vi "End Map.vi"   [LabVIEW 2017, in "LabPack.lvlib" / "Writer.lvclass"]
doc: "Finishes writing and encoding a series of key-value pairs (map) to MessagePack binary data format."
uses:
  Writer.lvclass
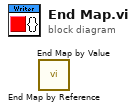
[diagram p0: block diagram]
diagram:
  n1 = call "End Map by Reference.vi"() -> ()  [unwired: 10 in, 2 out]
  n2 = call "End Map by Value.vi"() -> ()  [unwired: 10 in, 2 out]
